vi "LoadDev.vi"(6 "Path":path) -> (0 "ViStatus":T2, 1 "ModuleInfo":T4 {"DacScaleCoef" format="%#_2g"; "DacOffsetCoef" format="%#_2g"}, 3 "InterfaceInfo":T3)   [LabVIEW 2010]
panel:
  in  "step":T1(tab)
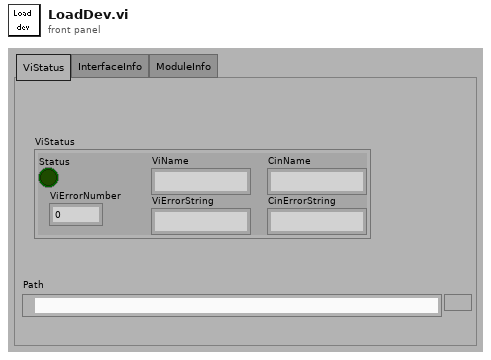
[diagram p1: front panel]
types:
  T1 = enum32{"ViStatus", "InterfaceInfo", "ModuleInfo"}
  T2 = cluster{"Status":bool, "ViErrorNumber":u32, "ViName":string, "ViErrorString":string, "CinName":string, "CinErrorString":string}
  T3 = cluster{"DllVersion":u32, "InterfaceType":u32, "InterfaceInstance":u32, "ModuleHandle":u32, "ReadBuffersParsArray":cluster{"Buffer":i16[], "ReadOv":u32, "ReadEvent":u32}[], "WriteBuffersParsArray":cluster{"Buffer":i16[], "WriteOv":u32, "WriteEvent":u32}[]}
  T4 = cluster{"VirtualSlot":u16, "ModuleName":string, "SerialNumber":string, "UsbSpeed":u8, "AvrVersion":string, "ModuleRevision":string, "DspType":string, "IsDacPresented":bool, "DspLoading":bool, "DspVersion":string, "DspClockout":u32, "AdcOffsetCoef":sgl[], "AdcScaleCoef":sgl[], "DacOffsetCoef":sgl[], "DacScaleCoef":sgl[]}
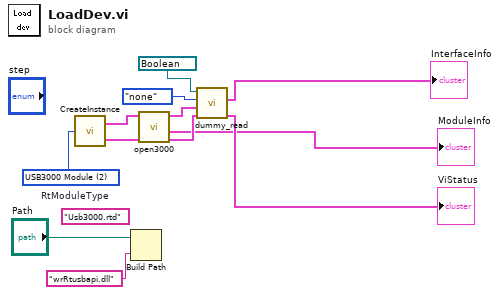
[diagram p0: block diagram]
diagram:
  w12 = u32 2 items=["Unknown Module", "USB2185 Module", "USB3000 Module"]  # RtModuleType
  (unwired) "Usb3000.rtd" ("DspDriverFile")
  n1 = call "CreateInstance.vi"("InterfaceType"=w12) -> ("InterfaceInfo"=w5:T3, "ViStatus"=w4:T2)
  n2 = Build Path(base path="Path", name or relative path="wrRtusbapi.dll" ("arg1")) -> ()  [unwired: 1 out]
  n3 = call "open3000.vi"("ViInfo"=w4, "InterfaceInfo"=w5) -> ("ViInfoOut"=w3:T2, "ModuleInfo"=→"ModuleInfo":T4, "InterfaceInfoOut"=w1:T3)  [unwired: 3 in]
  n4 = call "dummy_read.vi"("ViStatusOut 2"=w3, "InterfaceInfoOut 2"=w1, "SyncType3000"=enum16{"none", "TTL", "TTL_kadr", "analog"}."none", "Ctrl Reference"=refnum<vi> refnum) -> ("ViStatusOut"=→"ViStatus":T2, "InterfaceInfoOut"=→"InterfaceInfo":T3)  [unwired: 2 in]
